vi "UpdateSystemMessage.vi"(10 "Message":string, 11 "System Message Terminal Ref In":refnum<vi>) -> ()   [LabVIEW 2015]
doc: "Updates system message panel."
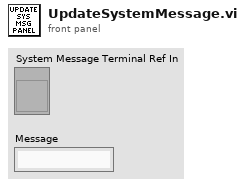
[diagram p1: front panel]
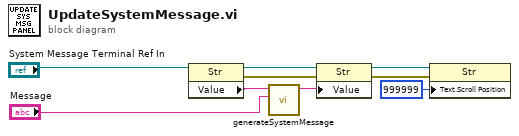
[diagram p0: block diagram]
diagram:
  n1 = property class="Str"(reference="System Message Terminal Ref In") -> (reference out=w8:refnum<vi>, error out=w9:errorcluster, "Value"=w5:string)  [unwired: 1 in]
  n2 = call "generateSystemMessage.vi"("New Message"="Message", "Old Message"=w5) -> ("System Message Output"=w7:string)  [unwired: 9 in]
  n3 = property class="Str"(reference=w8, error in=w9, "Value"=w7) -> (reference out=w3:refnum<vi>, error out=w2:errorcluster)
  n4 = property class="Str"(reference=w3, error in=w2, "Text.Scroll Position"=u32 999999) -> ()  [unwired: 2 out]
